vi "dlw_Modbus PLC.vi"(6 "Worker Alias":string="Modbus PLC", 7 "Caller in":refnum<class "Worker.lvclass">, 8 "error in":errorcluster, 10 "Initialization Data":T1, 11 "Modbus PLC in":refnum<class "Modbus PLC.lvclass">) -> (0 "error out":errorcluster, 3 "Modbus PLC out":refnum<class "Modbus PLC.lvclass">, 5 "dup Caller out":refnum<class "Worker.lvclass">)   [LabVIEW 2023, in "Modbus PLC.lvlib" / "Modbus PLC.lvclass"]
doc: "This VI dynamically loads the Worker that owns this VI as a subWorker into <b>Caller</b>, and returns the Worker's object containing the Worker's Public Properties. Initialization data that is to be received by this Worker's <Initialize> MHL case can be wired to <b>Initialization Data</b>. The dynamically loaded Worker requires an alias ( <b>Worker Alias</b> ) which must be unique to the Worker it is called from. If a currently loaded subWorker exists with the same Alias, an error will be returned.\n\n<b>Note:</b> This VI can only be used from <b>within</b> a Worker's MHL. To load this Worker from an external LabVIEW application or from TestStand, please use an Asynchronous Launcher VI.\n---"
uses:
  Modbus PLC.lvclass
  C:/Program Files/National Instruments/LabVIEW 2023/vi.lib/addons/_Workers/Library/Classes/Worker/Worker.lvclass
  <vilib>/addons/_Workers/Library/Classes/Worker/Worker.lvclass
  Initialization Data.ctl
  Response Cases.ctl
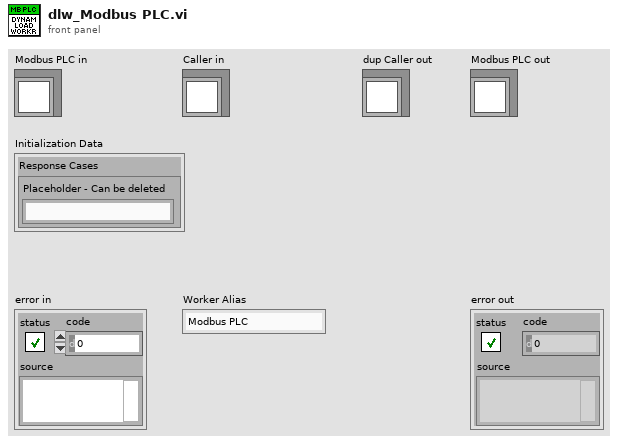
[diagram p1: front panel]
types:
  T1 = typedef "Modbus PLC.lvlib/Modbus PLC.lvclass/Initialization Data.ctl" = cluster{"Response Cases":T2}
  T2 = typedef "Modbus PLC.lvlib/Modbus PLC.lvclass/Response Cases.ctl" = cluster{"Placeholder - Can be deleted":string}
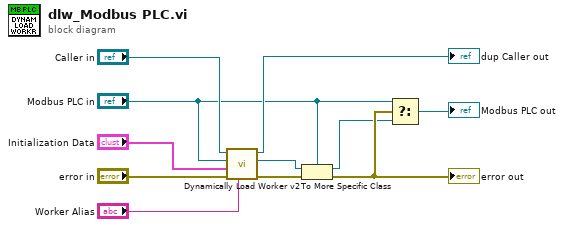
[diagram p0: block diagram]
diagram:
  n1 = call <vilib>:"Dynamically Load Worker v2.vi"("Worker Alias"="Worker Alias", "error in"="error in", "Initialization Data"="Initialization Data", "Worker to Dynamically Load"="Modbus PLC in", "Worker"="Caller in") -> ("error out"=w10:errorcluster, "Dynamically Loaded Worker out"=w5:refnum<class "Worker.lvclass">, "dup Worker out"=→"dup Caller out":refnum<class "Worker.lvclass">)  [unwired: 4 in]
  n2 = To More Specific Class(target class="Modbus PLC in", reference=w5, error in=w10) -> (specific class reference=w2:refnum<class "Modbus PLC.lvclass">, error out=w4:errorcluster)
  "error out" <- w4
  n3 = Select(t="Modbus PLC in", s=w4, f=w2) -> (s? t:f=→"Modbus PLC out":refnum<class "Modbus PLC.lvclass">)
